vi "Divide.vi"(8 "error in (no error)":errorcluster, 10 "input2":dbl, 11 "input1":dbl) -> (0 "error out":errorcluster, 2 "output":dbl)   [LabVIEW 2011]
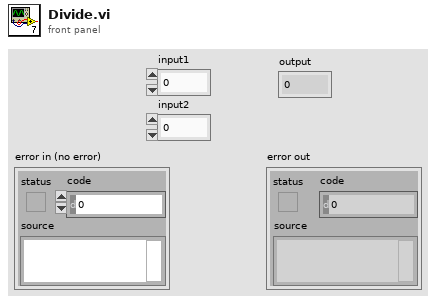
[diagram p1: front panel]
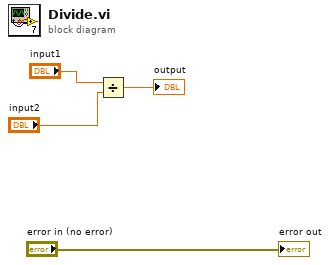
[diagram p0: block diagram]
diagram:
  n1 = Divide(x="input1", y="input2") -> (x/y=→"output":dbl)
  "error out" <- "error in (no error)"
